vi "sub_USRP_close_Rx.vi"(8 "Error in":errorcluster, 11 "Rx Session handle":refnum<k15>) -> (0 "Error out":errorcluster)   [LabVIEW 2012]
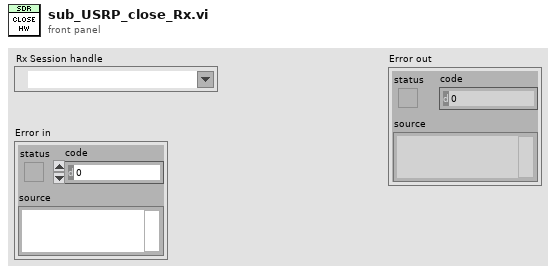
[diagram p1: front panel]
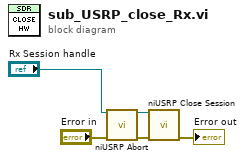
[diagram p0: block diagram]
diagram:
  n1 = call <instrlib>:"niUSRP Abort.vi"("session handle"="Rx Session handle", "error in (no error)"="Error in") -> ("session handle out"=w3:refnum<k15>, "error out"=w5:errorcluster)  [unwired: 12 in]
  n2 = call <instrlib>:"niUSRP Close Session.vi"("session handle"=w3, "error in (no error)"=w5) -> ("error out"=→"Error out":errorcluster)  [unwired: 13 in]
